vi "Write Audio History Buffer.vi"(10 "Audio History Buffer":dbl[][](array[numeric]), 11 "Effect Interface in":refnum<class "Effect Interface.lvclass">) -> (3 "Effect Interface out":refnum<class "Effect Interface.lvclass">)   [LabVIEW 2019, in "Effect Interface.lvlib" / "Effect Interface.lvclass"]
uses:
  Effect Interface.lvclass
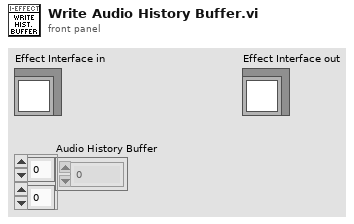
[diagram p1: front panel]
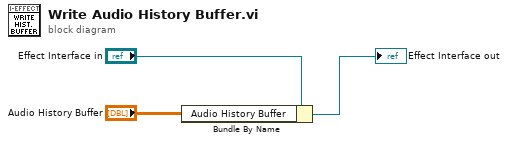
[diagram p0: block diagram]
diagram:
  n1 = Bundle By Name(cluster="Effect Interface in", "Audio History Buffer"="Audio History Buffer") -> (→"Effect Interface out":refnum<class "Effect Interface.lvclass">)
